vi "WriteFeatureList.vi"(6 "Feature Display Names":string[](array[string]), 7 "Feature Code Names":string[](array[string]), 8 "error in (no error)":errorcluster, 9 "Channel Name In":string, 10 "Group Name In":string, 11 "TDMS Ref In":refnum<k34>) -> (0 "error out":errorcluster, 1 "Channel Name Out":string, 2 "Group Name Out":string, 3 "TDMS Ref Out":refnum<k34>)   [LabVIEW 2017, in "Tdms.lvlib"]
uses:
  <vilib>/addons/InsightCM/Utilities/Tdms/Tdms.lvlib
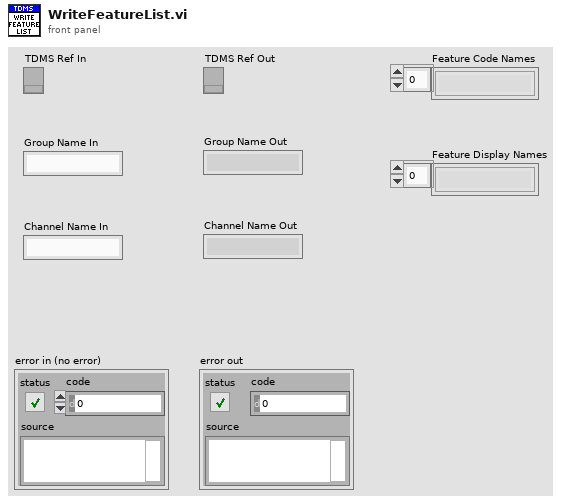
[diagram p1: front panel]
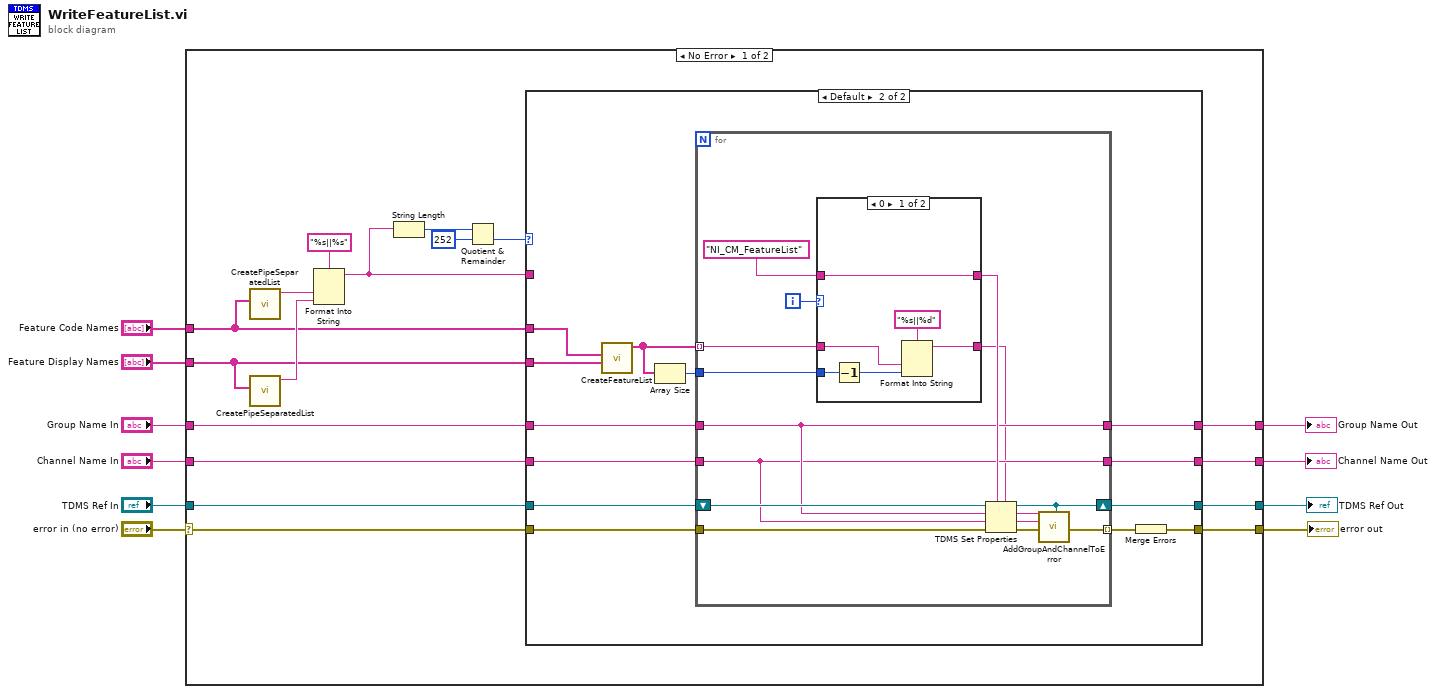
[diagram p0: block diagram]
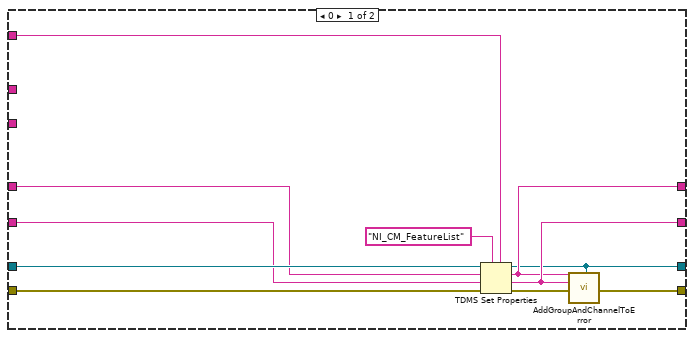
[diagram p2: hidden frame]
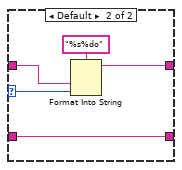
[diagram p3: hidden frame]
diagram:
  n1 = case shown="No Error" "error in (no error)" {
    selector: "error in (no error)" -> [w11 w81]
    tunnel: [w22 w81] -> w10
    tunnel: "TDMS Ref In" -> [w21 w80]
    tunnel: [w20 w80] -> w8
    tunnel: "Group Name In" -> [w18 w78]
    tunnel: [w17 w78] -> w6
    tunnel: "Channel Name In" -> [w16 w79]
    tunnel: [w15 w79] -> w4
    tunnel: "Feature Code Names" -> [w14 _]
    tunnel: "Feature Display Names" -> [w13 _]
    frame No Error {
      n2 = call <vilib>:"CreatePipeSeparatedList.vi"("Array"=w14) -> ("List Out"=w26:string)  [unwired: 10 in]
      n3 = call <vilib>:"CreatePipeSeparatedList.vi"("Array"=w13) -> ("List Out"=w25:string)  [unwired: 10 in]
      n4 = Format Into String(format string="%s||%s", w26, w25) -> (resulting string=w19:string)  [unwired: 2 in, 1 out]
      n5 = String Length(string=w19) -> (length=w24:i32)
      n6 = Quotient & Remainder(x=w24, y=252) -> (floor(x/y)=w12:i32)  [unwired: 1 out]
      n7 = case shown="Default" w12 {
        tunnel: w11 -> [w38 w49]
        tunnel: [w31 w43] -> w22
        tunnel: w21 -> [w37 w46]
        tunnel: [w28 w45] -> w20
        tunnel: w19 -> [w36 _]
        tunnel: w18 -> [w34 w48]
        tunnel: [w29 w42] -> w17
        tunnel: w16 -> [w33 w47]
        tunnel: [w30 w41] -> w15
        tunnel: w14 -> [_ w50]
        tunnel: w13 -> [_ w51]
        frame 0 {
          n8 = TDMS Set Properties(5:w36, 7:"NI_CM_FeatureList" ("property names"), 8:w38, 9:w33, 10:w34, 11:w37) -> (0:w32:errorcluster, 1:w30:string, 2:w29:string, 3:w28:refnum<k34>)
          n9 = call <vilib>:"AddGroupAndChannelToError.vi"("error in (no error)"=w32, "channel name in"=w30, "group name in"=w29, "Refnum in"=w28) -> ("error out"=w31:errorcluster)  [unwired: 15 in]
        }
        frame Default {
          n10 = call <vilib>:"CreateFeatureList.vi"("feature display names"=w51, "feature code names"=w50) -> ("feature lists"=w40:string[])  [unwired: 9 in]
          n11 = Array Size(array=w40) -> (size(s)=w39:i32)
          n12 = for {
            tunnel: w40 -> [w54] mode=indexing
            shift-right: [w56] -> w45
            shift-left: w46 -> [w64]
            tunnel: w49 -> [w65]
            tunnel: [w59] -> w44 mode=indexing
            tunnel: w48 -> [w62]
            tunnel: w47 -> [w61]
            tunnel: [w62] -> w42
            tunnel: [w61] -> w41
            tunnel: w39 -> [w53]
            i -> [w52]
            n13 = case shown="0" w52 {
              selector: w52 -> [_ w73]
              tunnel: "NI_CM_FeatureList" ("property name") -> [w72 w76]
              tunnel: [w72 w74] -> w63
              tunnel: [w67 w75] -> w55
              tunnel: w54 -> [w68 w75]
              tunnel: w53 -> [w71 _]
              frame 0 {
                n14 = Decrement(x=w71) -> (x-1=w69:i32)
                n15 = Format Into String(format string="%s||%d", w68, w69) -> (resulting string=w67:string)  [unwired: 2 in, 1 out]
              }
              frame Default {
                n16 = Format Into String(format string="%s%do", w76, w73) -> (resulting string=w74:string)  [unwired: 2 in, 1 out]
              }
            }
            n17 = TDMS Set Properties(5:w55, 7:w63, 8:w65, 9:w61, 10:w62, 11:w64) -> (0:w60:errorcluster, 1:w58:string, 2:w57:string, 3:w56:refnum<k34>)
            n18 = call <vilib>:"AddGroupAndChannelToError.vi"("error in (no error)"=w60, "channel name in"=w58, "group name in"=w57, "Refnum in"=w56) -> ("error out"=w59:errorcluster)  [unwired: 15 in]
          }
          n19 = Merge Errors(w44) -> (w43:errorcluster)
        }
      }
    }
    frame Error {
    }
  }
  "Channel Name Out" <- w4
  "Group Name Out" <- w6
  "TDMS Ref Out" <- w8
  "error out" <- w10
